vi "TestClone.vi"() -> ()   [LabVIEW 2014, in "WfrmModule.lvlib"]
uses:
  WfrmModule.lvlib
  WfrmPlugins/EventPluginBaseClass/TypeDefs/WfrmConfig.ctl
  PublicAPI/Arguments/Requests/dblEvtParams.ctl
  PublicAPI/Arguments/Requests/dblTimeArray.ctl
  WfrmPlugins/EventPluginBaseClass/TypeDefs/clEvtReportArray.ctl
  WfrmPlugins/EventPluginBaseClass/TypeDefs/clEvtReport.ctl
  WfrmPlugins/EventPluginBaseClass/TypeDefs/dblEvtSignalArray.ctl
  PublicAPI/Arguments/Requests/clTimeParams.ctl
  <userlib>/NIST/ModuleAdminLib/ModuleAdmin/ModuleAdmin.lvclass/ModuleAdmin.ctl
  <userlib>/NIST/ModuleAdminLib/ModuleAdmin/ModuleAdmin.lvclass
  WfrmPlugins/EventPluginBaseClass/TypeDefs/clWfrmParams.ctl
  PublicAPI/Arguments/Broadcasts/clDidInit.ctl
  PublicAPI/Arguments/Requests/clStopArgument.ctl
  <userlib>/NIST/ModuleAdminLib/ModuleAdmin/Accessors/Read CloneRegRef.vi
  <userlib>/NIST/ModuleAdminLib/ModuleAdmin/Accessors/Write CloneRegRef.vi
  <userlib>/NIST/ModuleAdminLib/CloneRegistration/CloneRegistration.lvclass
  WfrmPlugins/EventPluginBaseClass/BaseWfrmPlugin.lvclass
  <vilib>/Analysis/NI_AALBase.lvlib
  <vilib>/Analysis/1siggen.llb/Ramp Pattern by Delta.vi
panel:
  in  "btnConfigure":bool
  out "Settling Time":dbl
  in  "End Time":dbl=10.0
  in  "Start Time":dbl
  in  "WfrmParams":string[][](table)
  in  "Plugin Type":u16(ring) items=["C37.118.1", "HIL PMU", "60255Harm", "User1", "User2"]
  in  "clTimeParams":T1={"dblTimeArray"=[0.0, 0.05, 0.1, 0.15000000000000002, 0.2], "StartTime"=0.0, "EndTime"=1.0, "SettlingTime"=0.0}
  in  "btnSendArbWfrm":bool
  in  "btnGetEvtSignal":bool
  out "dblEventSignalArray":T2
  out "PathToPluginIniFileReport":path=path "P:/Framework/Events/EventPlugins/SSEvtPlugin/SteadyStateEventPlugin.ini"
  in  "btnReadPathToPlugin":bool
  in  "btnGetEvtReportArray":bool
  out "clEvtReportArray":T3 {"Synx" format="%#_4g"}
  in  "btnReadEvtParams":bool
  in  "btnWriteEvtParams":bool
  in  "btnReadTimeArray":bool
  in  "btnWriteTimeArray":bool
  out "dblTimeArrayReport":T5
  out "dblEvtParamsReport":T6
  in  "btnReadEvtConfig":bool
  in  "clEvtConfig":T7={"T0(UTC)"=0.0, "F0"=60.0, "Fs"=60, "FSamp"=960}
  in  "btnWriteEvtConfig":bool
  in  "btnLoadPlugin":bool
  in  "btnRemove":bool
  out "Status":string
  out "Active Modules (Array)":string[](array[string])
  in  "btnAdd":bool
  in  "btnStop":bool
  in  "Select Module":i32(ring)=-1 caption="Select Module to send Request" items=["All"=-1, "4140002"=4140002]
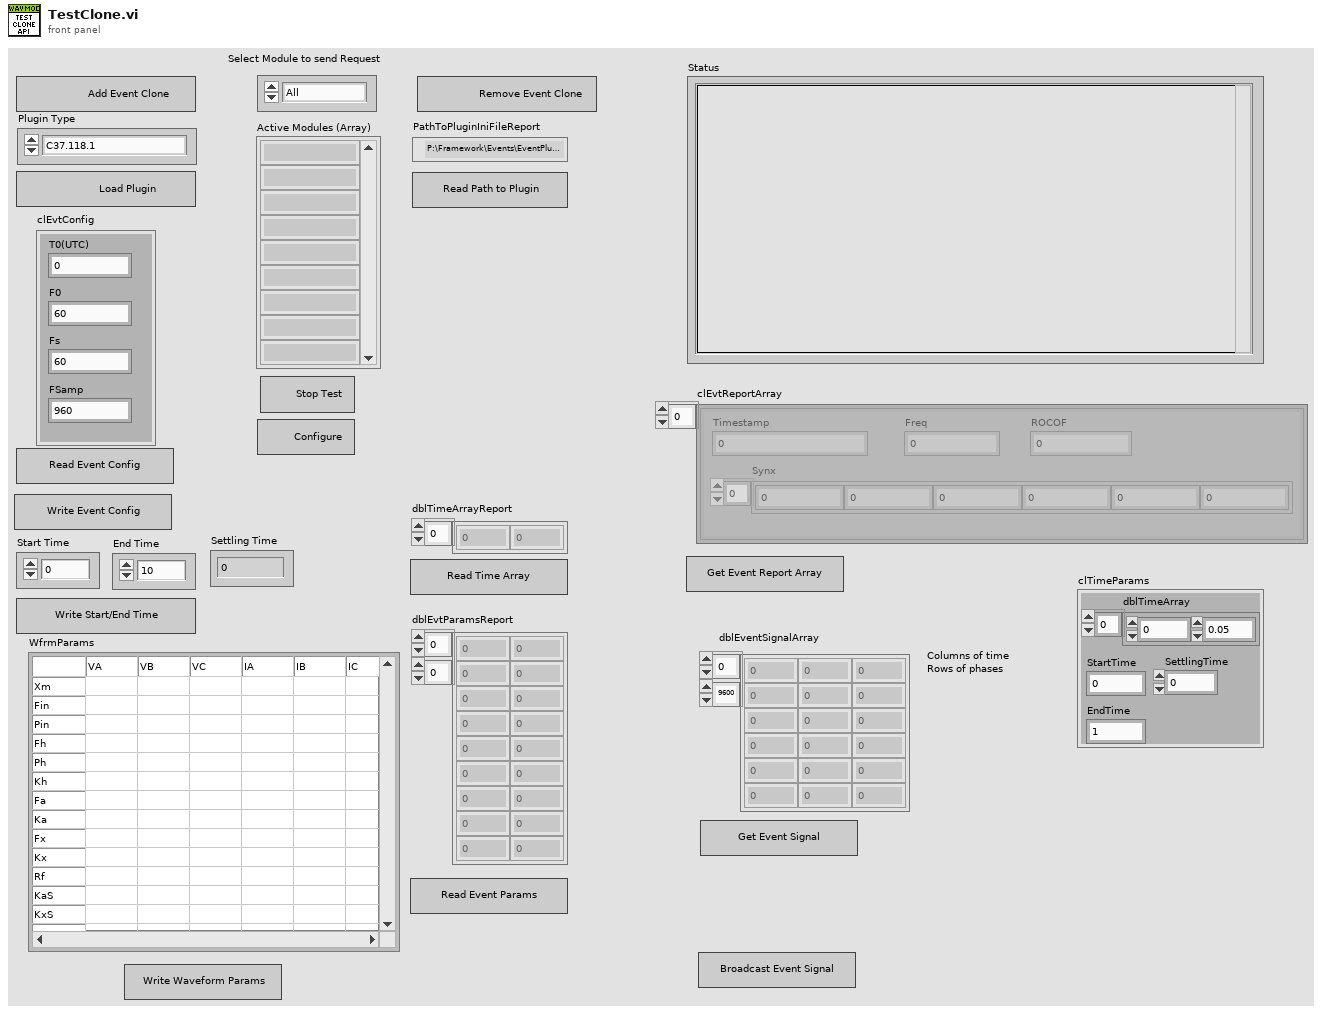
[diagram p1: front panel]
types:
  T1 = typedef "WfrmModule.lvlib/clTimeParams.ctl" = cluster{"dblTimeArray":dbl[], "StartTime":dbl, "EndTime":dbl, "SettlingTime":dbl}
  T2 = typedef "WfrmPlugins.lvlib/BaseWfrmPlugin.lvclass/dblEvtSignalArray.ctl" = dbl[][]
  T3 = typedef "WfrmPlugins.lvlib/BaseWfrmPlugin.lvclass/clEvtReportArray.ctl" = T4[]
  T4 = typedef "WfrmPlugins.lvlib/BaseWfrmPlugin.lvclass/clEvtReport.ctl" = cluster{"Timestamp":dbl, "Synx":cdb[], "Freq":dbl, "ROCOF":dbl}
  T5 = typedef "WfrmModule.lvlib/dblTimeArray.ctl" = dbl[]
  T6 = typedef "WfrmModule.lvlib/dblEvtParams.ctl" = dbl[][]
  T7 = typedef "WfrmPlugins.lvlib/BaseWfrmPlugin.lvclass/WfrmConfig.ctl" = cluster{"T0(UTC)":dbl, "F0":dbl, "Fs":i32, "FSamp":u32}
  T8 = typedef "WfrmModule.lvlib/clBroadcastEvents.ctl" = cluster{"DidInit":refnum<user-event>, "StatusUpdate":refnum<user-event>, "ErrorReport":refnum<user-event>, "DidStop":refnum<user-event>, "ReadEvtConfig":refnum<user-event>, "ReadTimeArray":refnum<user-event>, "ReadEvtParams":refnum<user-event>, "GetEvtReportArray":refnum<user-event>, "ReadPathToPlugin":refnum<user-event>, "GetEvtSignal":refnum<user-event>, "SendArbWfrm":refnum<user-event>, "WfrmParams":refnum<user-event>, "StartEndSettling":refnum<user-event>}
  T9 = typedef "WfrmPlugins.lvlib/BaseWfrmPlugin.lvclass/clWfrmParams.ctl" = cluster{"RowHdrs":string[], "ColHdrs":string[], "DefaultParams":string[][]}
  T10 = typedef "WfrmModule.lvlib/clDidInit.ctl" = cluster{"Init?":bool, "ModuleAdmin":refnum<class "ModuleAdmin.lvclass">}
  T11 = typedef "WfrmModule.lvlib/clStopArgument.ctl" = cluster{"Exit via Stop Module Req?":bool, "Wait for Module to stop?":bool, "ModuleAdmin":refnum<class "ModuleAdmin.lvclass">}
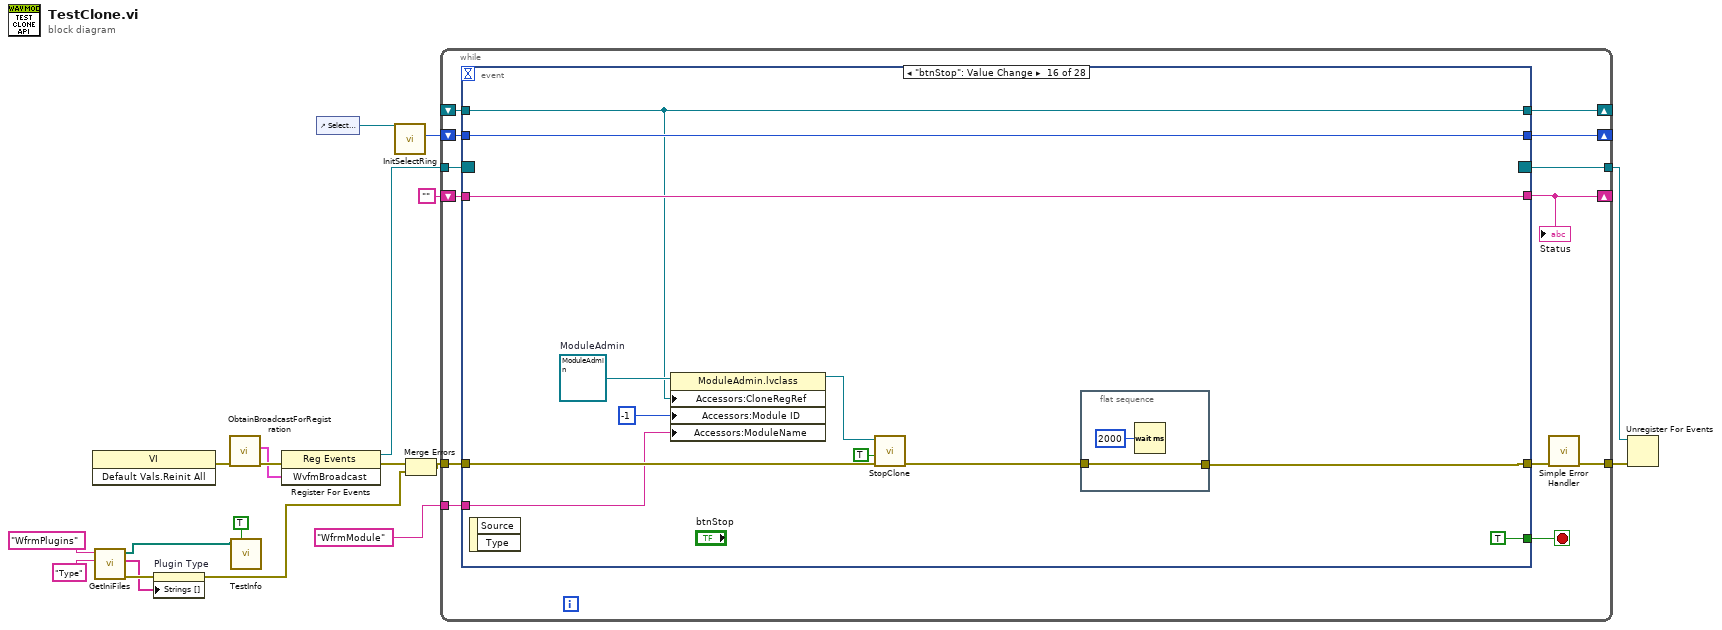
[diagram p0: block diagram]
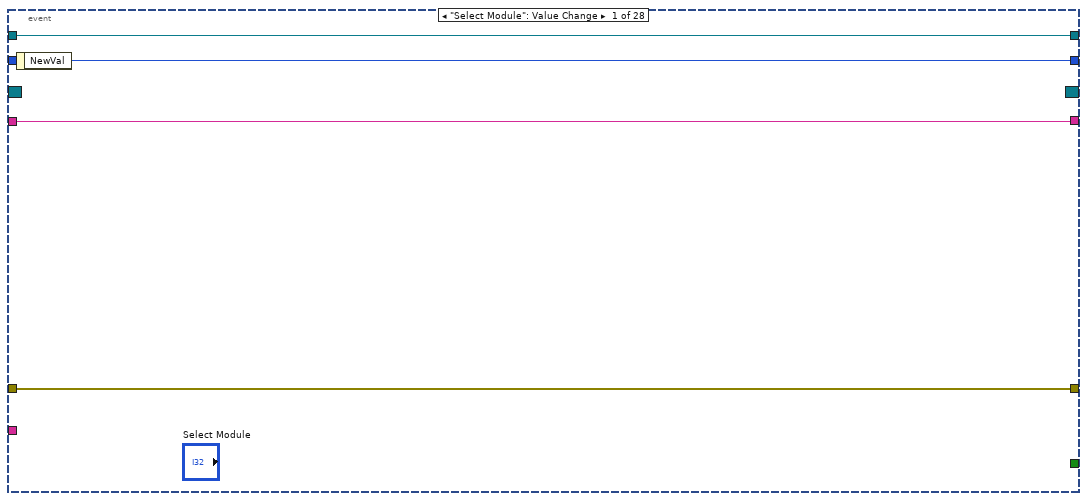
[diagram p2: hidden frame]
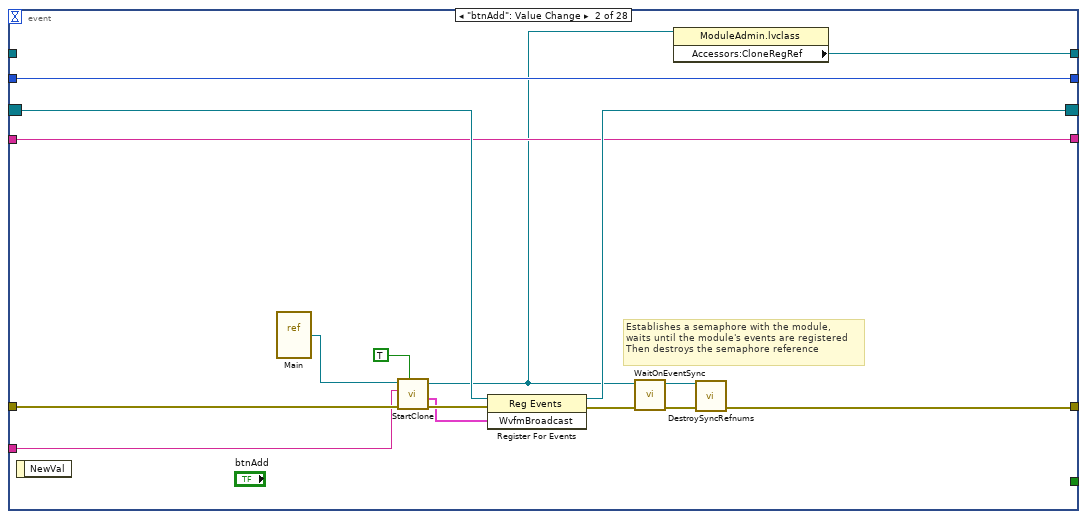
[diagram p3: hidden frame]
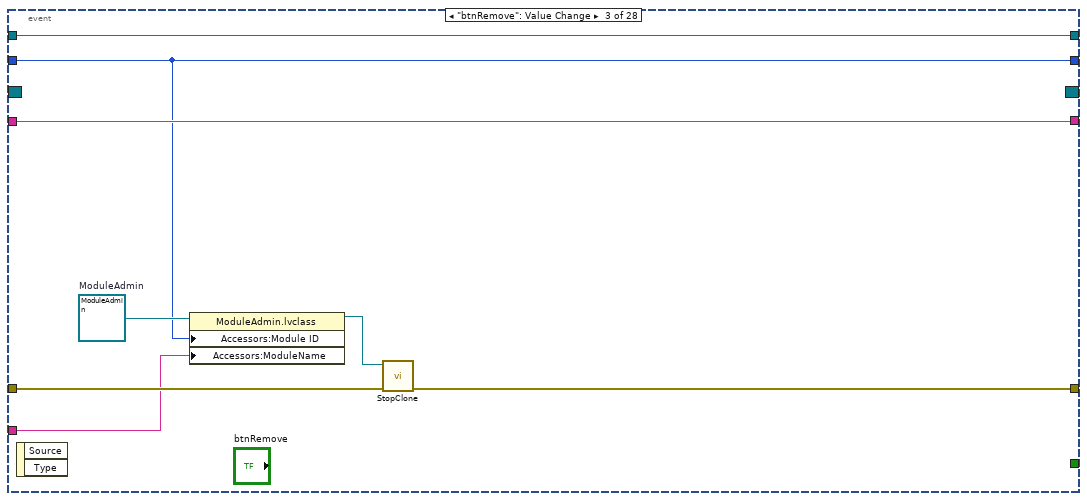
[diagram p4: hidden frame]
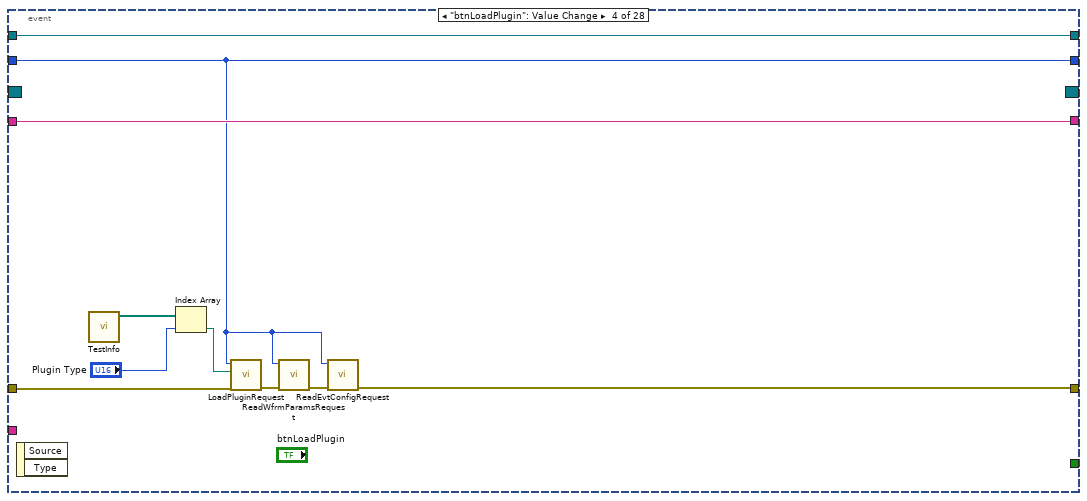
[diagram p5: hidden frame]
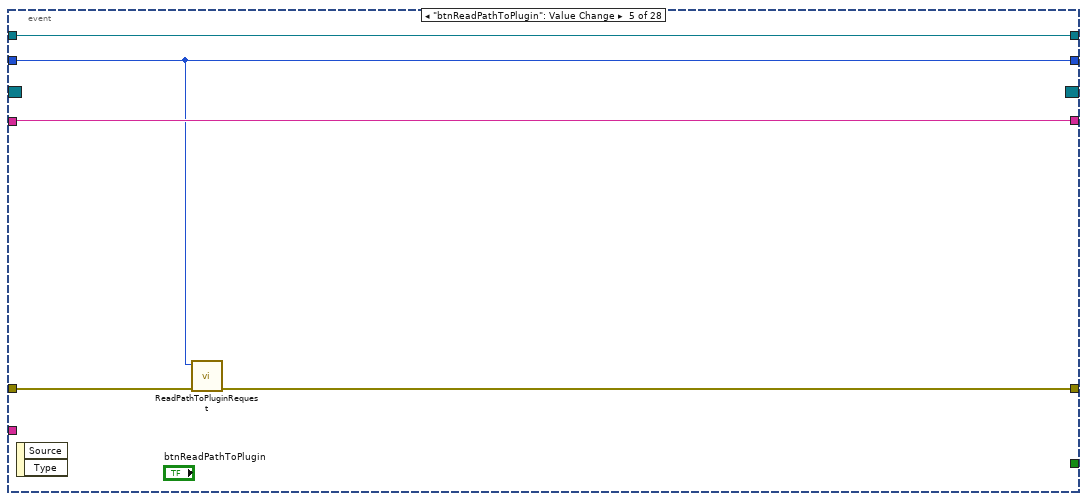
[diagram p6: hidden frame]
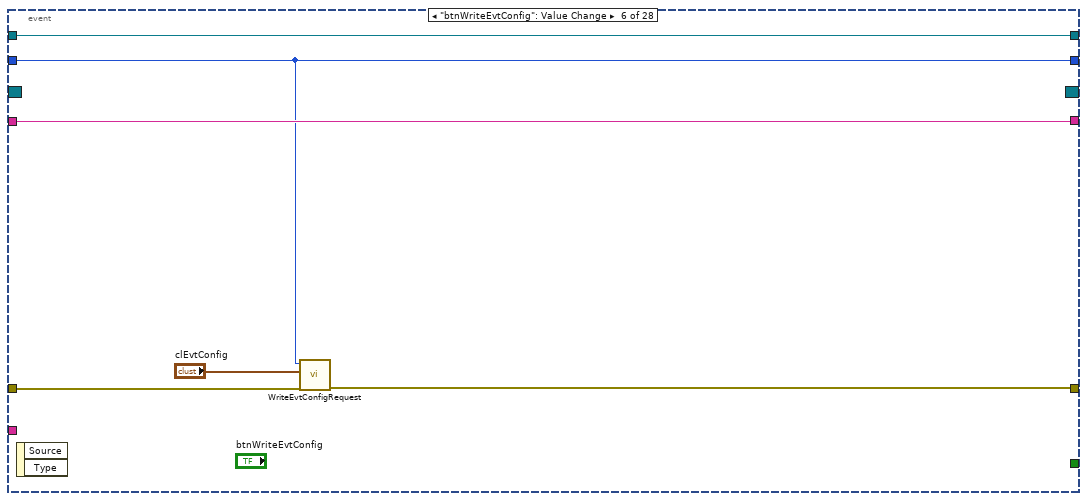
[diagram p7: hidden frame]
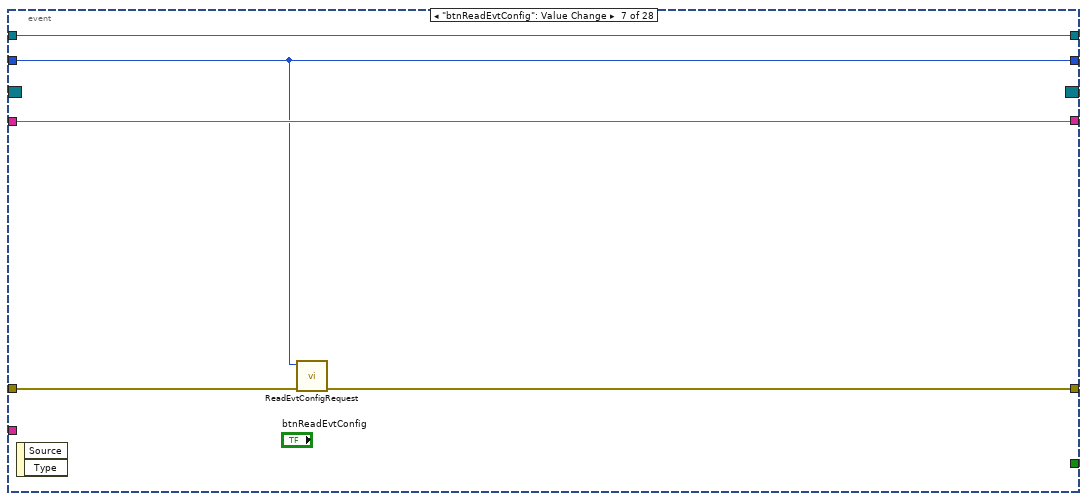
[diagram p8: hidden frame]
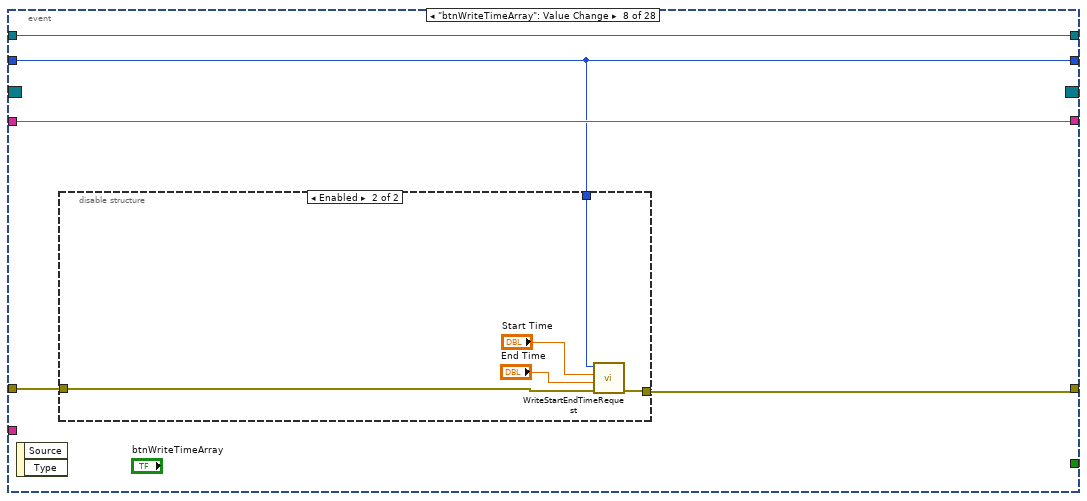
[diagram p9: hidden frame]
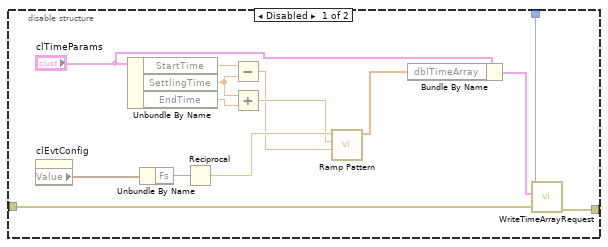
[diagram p10: hidden frame]
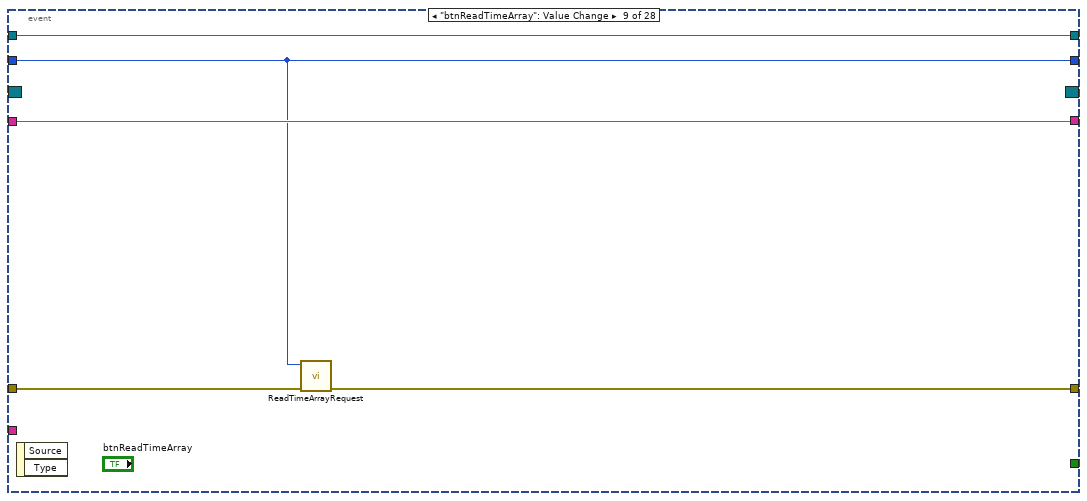
[diagram p11: hidden frame]
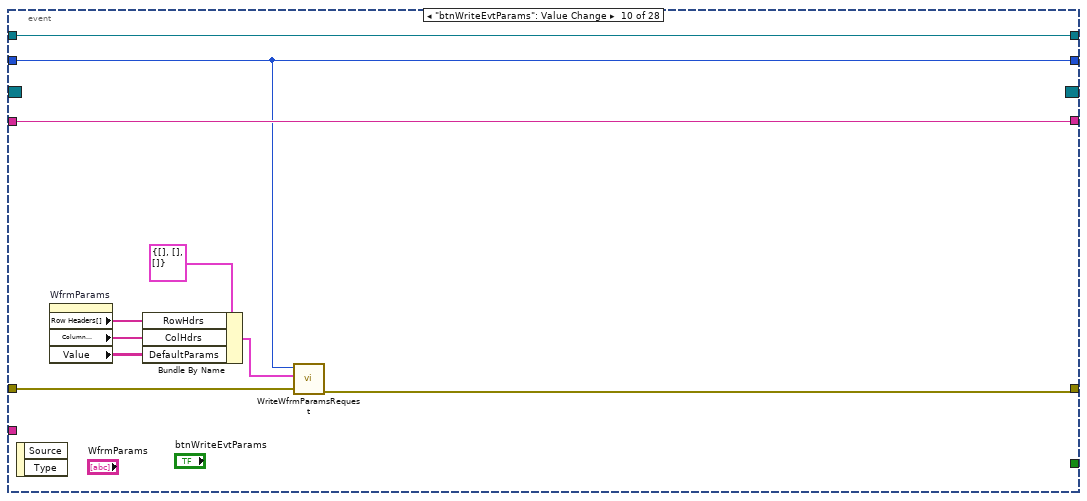
[diagram p12: hidden frame]
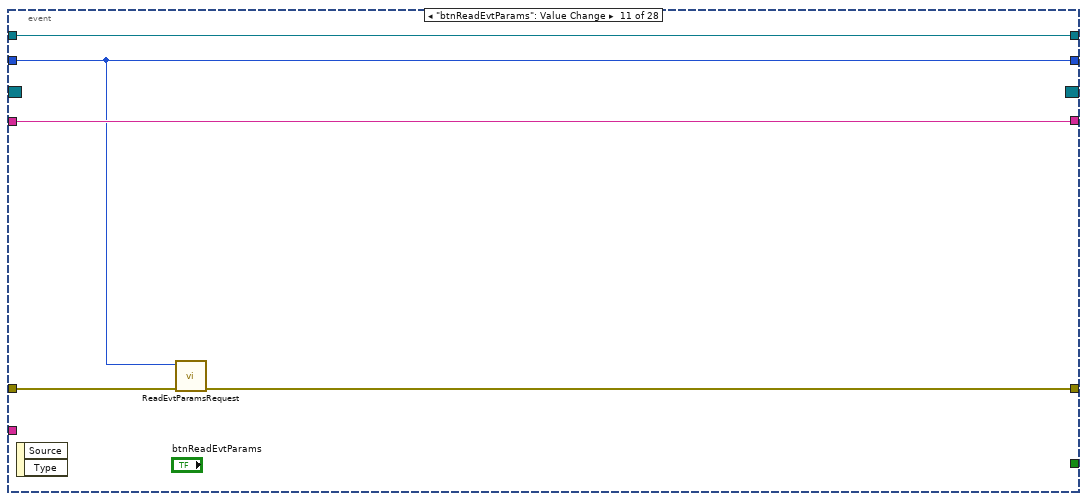
[diagram p13: hidden frame]
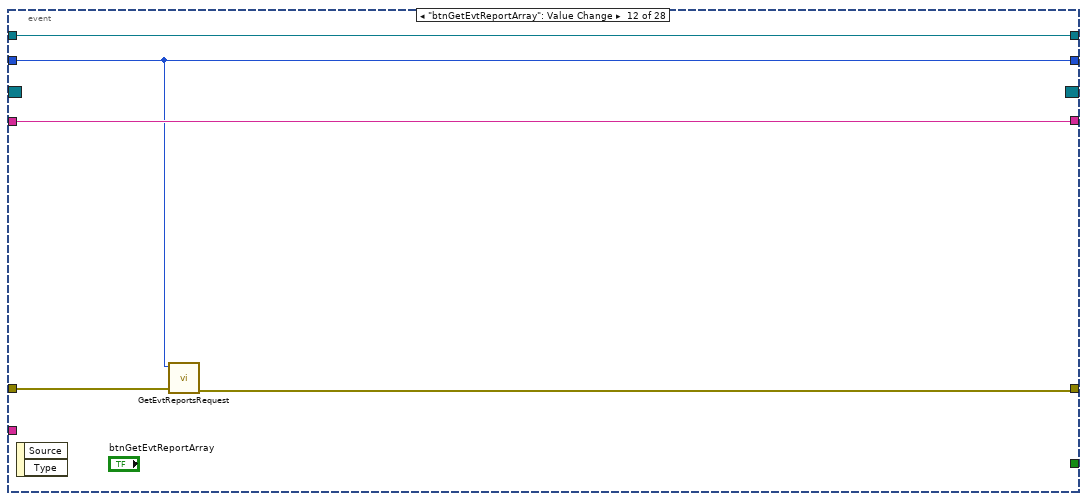
[diagram p14: hidden frame]
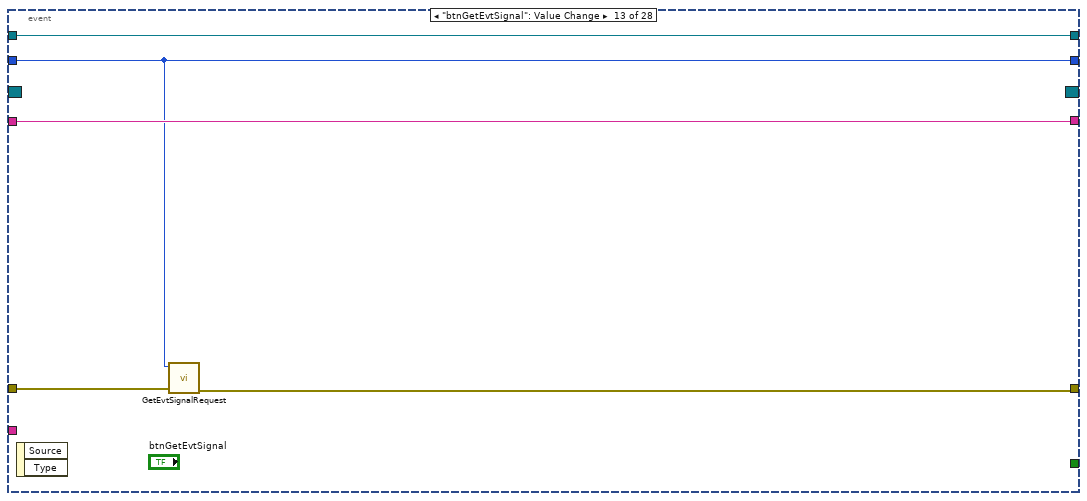
[diagram p15: hidden frame]
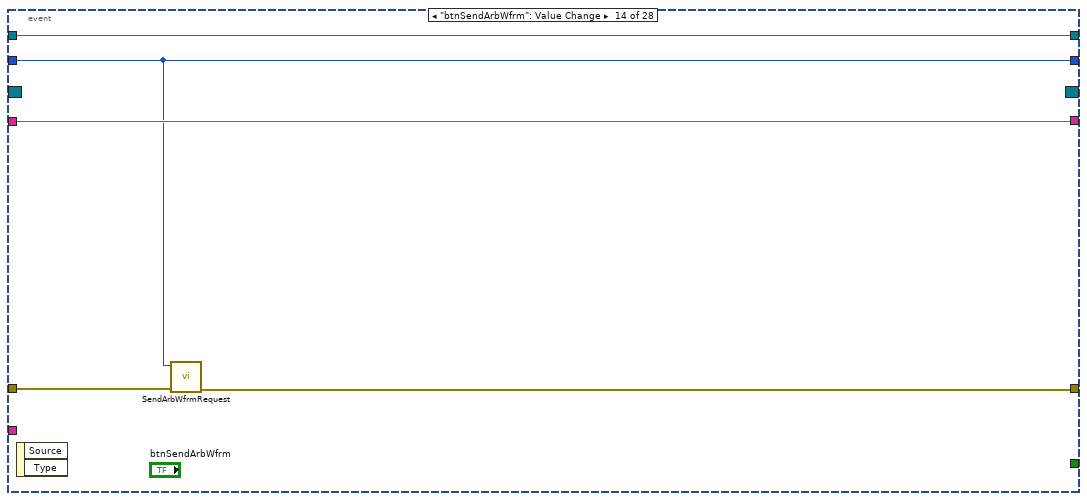
[diagram p16: hidden frame]
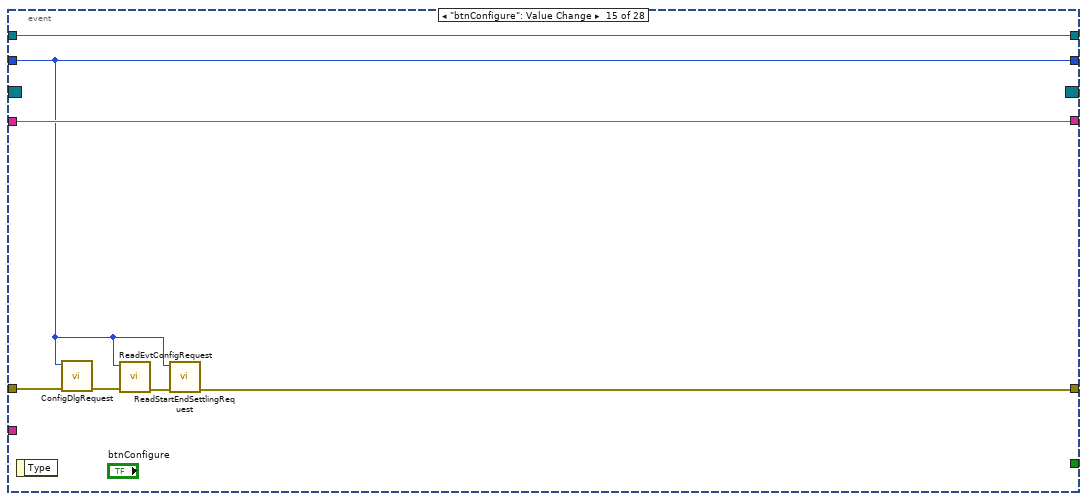
[diagram p17: hidden frame]
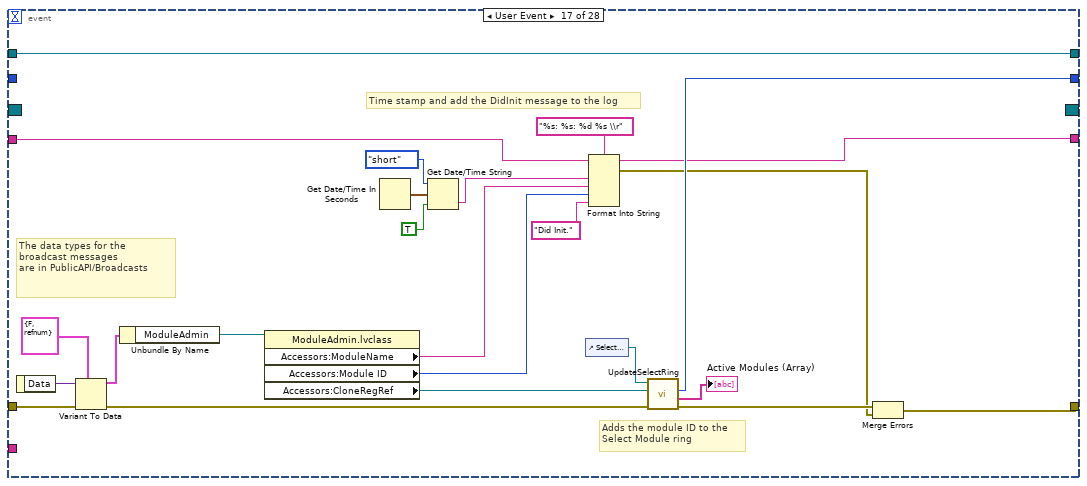
[diagram p18: hidden frame]
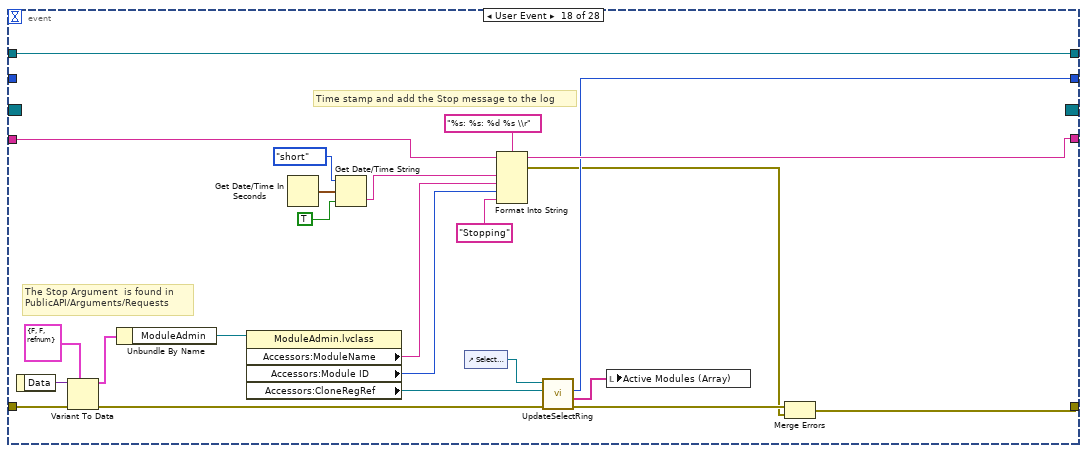
[diagram p19: hidden frame]
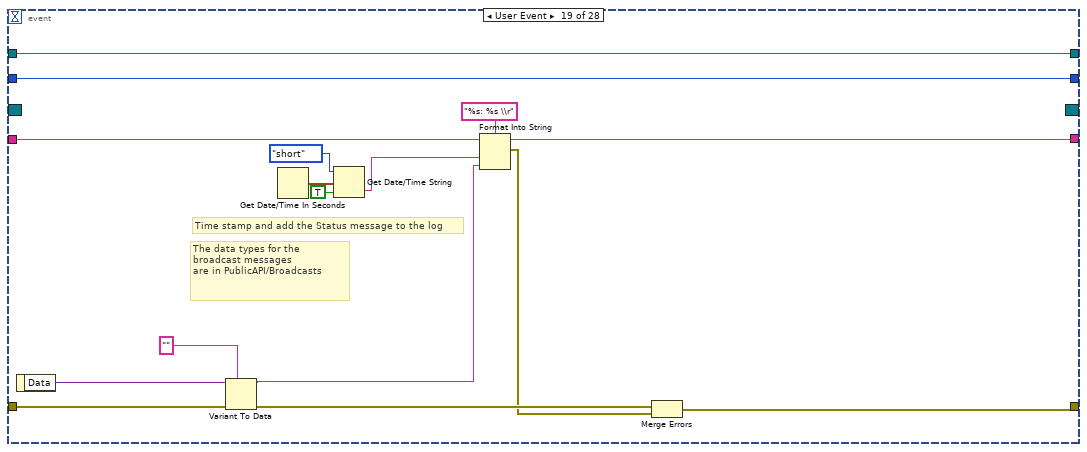
[diagram p20: hidden frame]
diagram:
  n1 = invoke class="VI" method="Default Vals.Reinit All"() -> (error out=w17:errorcluster)  [unwired: 3 in, 2 out]
  n2 = call "GetIniFiles.vi"("iniKey"="Type", "name or relative path"="WfrmPlugins") -> ("error out"=w10:errorcluster, "Types"=w9:string[], "IniFilePaths"=w5:path[])  [unwired: 7 in]
  n3 = property on="Plugin Type" class="Ring (strict)"(error in=w10, "Strings []"=w9) -> (error out=w7:errorcluster)  [unwired: 1 in, 1 out]
  n4 = call "ObtainBroadcastForRegistration.vi"("error in (no error)"=w17) -> ("error out"=w16:errorcluster, "WvfmBroadcast"=w15:T8)  [unwired: 9 in]
  n5 = call "TestInfo.vi"("Set (f)"=TRUE, "PluginIniFilePaths"=w5) -> ()  [unwired: 9 in, 1 out]
  n6 = register-events(error in=w16, w15) -> (reference out=w13:refnum<event-registration>, error out=w14:errorcluster)  [unwired: 1 in]
  n7 = control-ref of="Select Module"() -> (w19:refnum<vi>)
  n8 = call "InitSelectRing.vi"("Ring Refnum"=w19) -> ("Module Ring Value"=w18:i32)  [unwired: 9 in, 1 out]
  n9 = Merge Errors(w14, w7) -> (w8:errorcluster)
  n10 = while {
    shift-right: [w31] -> _
    shift-left: w18 -> [w32]
    tunnel: w8 -> [w29]
    tunnel: w13 -> [w26]
    tunnel: [w27] -> w2
    shift-right: [w25] -> _
    shift-left: "" -> [w24]
    tunnel: "WfrmModule" ("ModuleName") -> [w23]
    tunnel: [w22] -> w1
    shift-right: [w21] -> _
    shift-left: _ -> [w20]
    stop <- w30 stop-if-true
    n11 = event shown="[15] \"btnStop\": Value Change" {
      selector: w26 -> [_ w44 _ _ _ _ _ _ _ _ _ _ _ _ _ _ _ _ _ _ _ _ _ _ _ _ _ _]
      dyn-events: [_ w43 _ _ _ _ _ _ _ _ _ _ _ _ _ _ _ _ _ _ _ _ _ _ _ _ _ _] -> w22
      timeout: _ -> [_ _ _ _ _ _ _ _ _ _ _ _ _ _ _ _ _ _ _ _ _ _ _ _ _ _ _ _]
      tunnel: w32 -> [_ w52 w55 w61 w71 w77 w82 w87 w113 w121 w127 w131 w136 w141 w146 w163 _ _ w229 w234 w244 w251 w259 w266 w280 w287 w296 w312]
      tunnel: [w36 w52 w55 w61 w71 w77 w82 w87 w113 w121 w127 w131 w136 w141 w146 w163 w184 w200 w229 w234 w244 w251 w259 w266 w280 w287 w296 w312] -> w31
      tunnel: [_ _ _ _ _ _ _ _ _ _ _ _ _ _ _ TRUE _ _ _ _ _ _ _ _ _ _ _ _] -> w30
      tunnel: w29 -> [w34 w51 w59 w69 w73 w79 w84 w90 w112 w124 w128 w134 w139 w143 w151 w161 w189 w209 w226 w238 w246 w256 w261 w275 w283 w292 w300 w310]
      tunnel: [w34 w45 w58 w62 w72 w76 w83 w89 w111 w122 w126 w133 w138 w142 w145 w154 w172 w197 w220 w237 w240 w255 w262 w268 w282 w291 w299 w303] -> w28
      tunnel: [w35 w41 w60 w68 w74 w80 w85 w88 w114 w123 w129 w132 w137 w144 w149 w159 w176 w206 w223 w233 w245 w250 w260 w265 w281 w288 w297 w307] -> w25
      tunnel: w24 -> [w35 w41 w60 w68 w74 w80 w85 w88 w114 w123 w129 w132 w137 w144 w149 w159 w175 w207 w228 w233 w245 w250 w260 w265 w281 w288 w297 w307]
      tunnel: w23 -> [_ w40 w56 _ _ _ _ _ _ _ _ _ _ _ _ w157 _ _ _ _ _ _ _ _ _ _ _ _]
      tunnel: [w33 w37 w53 w64 w70 w75 w81 w86 w110 w120 w125 w130 w135 w140 w150 w152 w166 w190 w214 w230 w243 w249 w257 w267 w277 w285 w293 w313] -> w21
      tunnel: w20 -> [w33 _ w53 w64 w70 w75 w81 w86 w110 w120 w125 w130 w135 w140 w150 w152 w166 w190 w214 w230 w243 w249 w257 w267 w277 w285 w293 w313]
      event "Select Module": Value Change {
        n12 = event-data() -> ("NewVal"=w36:i32)  [unwired: 1 in]
      }
      event "btnAdd": Value Change {
        # "Establishes a semaphore with the module,\nwaits until the module's events are registered\nThen destroys the semaphore reference"
        n13 = event-data() -> ()  [unwired: 1 in, 1 out]
        n14 = vi-ref "Main.vi"() -> (w42:refnum<vi>)
        n15 = call "StartClone.vi"("ShowPanel? (F)"=TRUE, "error in (no error)"=w51, "ModuleName"=w40, "VI Refnum"=w42) -> ("error out"=w50:errorcluster, "WvfrmEvents"=w46:T8, "ModuleAdmin"=w38:refnum<class "ModuleAdmin.lvclass">)  [unwired: 5 in]
        n16 = register-events(reference=w44, error in=w50, w46) -> (reference out=w43:refnum<event-registration>, error out=w49:errorcluster)
        n17 = call <userlib>:"WaitOnEventSync.vi"("error in (no error)"=w49, "ModuleAdmin"=w38) -> ("error out"=w48:errorcluster, "ModuleAdmin"=w47:refnum<class "ModuleAdmin.lvclass">)  [unwired: 8 in]
        n18 = property class="ModuleAdmin.lvclass"(reference=w38) -> ("Accessors:CloneRegRef"=w37:refnum<data-value>)  [unwired: 1 in, 2 out]
        n19 = call <userlib>:"DestroySyncRefnums.vi"("error in (no error)"=w48, "ModuleAdmin"=w47) -> ("error out"=w45:errorcluster)  [unwired: 9 in]
      }
      event "btnRemove": Value Change {
        w57 = refnum<class "ModuleAdmin.lvclass"> refnum  # ModuleAdmin
        n20 = event-data() -> ()  [unwired: 1 in, 2 out]
        n21 = property class="ModuleAdmin.lvclass"(reference=w57, "Accessors:Module ID"=w55, "Accessors:ModuleName"=w56) -> (reference out=w54:refnum<class "ModuleAdmin.lvclass">)  [unwired: 1 in, 1 out]
        n22 = call "StopClone.vi"("error in (no error)"=w59, "ModuleAdmin"=w54) -> ("error out"=w58:errorcluster)  [unwired: 9 in]
      }
      event "btnLoadPlugin": Value Change {
        n23 = event-data() -> ()  [unwired: 1 in, 2 out]
        n24 = call "TestInfo.vi"() -> ("PluginIniFilePaths"=w67:path[])  [unwired: 11 in]
        n25 = Index Array(array=w67, index="Plugin Type") -> (element=w65:path)
        n26 = call "LoadPluginRequest.vi"("error in (no error)"=w69, "PathToPlugin"=w65, "ModuleID"=w61) -> ("error out"=w63:errorcluster)  [unwired: 8 in]
        n27 = call "ReadWfrmParamsRequest.vi"("error in (no error)"=w63, "ModuleID"=w61) -> ("error out"=w62:errorcluster)  [unwired: 9 in]
        n28 = call "ReadEvtConfigRequest.vi"("error in (no error)"=w62, "ModuleID"=w61) -> ()  [unwired: 9 in, 1 out]
      }
      event "btnReadPathToPlugin": Value Change {
        n29 = event-data() -> ()  [unwired: 1 in, 2 out]
        n30 = call "ReadPathToPluginRequest.vi"("error in (no error)"=w73, "ModuleID"=w71) -> ("error out"=w72:errorcluster)  [unwired: 9 in]
      }
      event "btnWriteEvtConfig": Value Change {
        n31 = event-data() -> ()  [unwired: 1 in, 2 out]
        n32 = call "WriteEvtConfigRequest.vi"("error in (no error)"=w79, "clEvtConfig"="clEvtConfig", "ModuleID"=w77) -> ("error out"=w76:errorcluster)  [unwired: 8 in]
      }
      event "btnReadEvtConfig": Value Change {
        n33 = event-data() -> ()  [unwired: 1 in, 2 out]
        n34 = call "ReadEvtConfigRequest.vi"("error in (no error)"=w84, "ModuleID"=w82) -> ("error out"=w83:errorcluster)  [unwired: 9 in]
      }
      event "btnWriteTimeArray": Value Change {
        n35 = event-data() -> ()  [unwired: 1 in, 2 out]
        n36 = disable-structure shown="Enabled" {
          disable-tunnel: w90 -> [w104 w109]
          disable-tunnel: [w103 w108] -> w89
          disable-tunnel: w87 -> [w102 w106]
          frame Disabled {
            n37 = property on="clEvtConfig" class="Clust (strict)"() -> ("Value"=w101:T7)  [unwired: 2 in, 2 out]
            n38 = Unbundle By Name("clTimeParams") -> ("StartTime"=w98:dbl, "SettlingTime"=w97:dbl, "EndTime"=w96:dbl)
            n39 = Unbundle By Name(w101) -> ("Fs"=w100:i32)
            n40 = Reciprocal(x=w100) -> (1/x=w99:dbl)
            n41 = Subtract(x=w98, y=w97) -> (x-y=w94:dbl)
            n42 = Add(x=w97, y=w96) -> (x+y=w95:dbl)
            n43 = call-poly <vilib>:"Ramp Pattern.vi"("start"=w94, "end"=w95, "delta"=w99) -> ("Ramp Pattern"=w92:dbl[])  [unwired: 6 in, 2 out]
            n44 = Bundle By Name(cluster="clTimeParams", "dblTimeArray"=w92) -> (w91:T1)
            n45 = call "WriteTimeArrayRequest.vi"("error in (no error)"=w104, "clTimeParams"=w91, "ModuleID"=w102) -> ("error out"=w103:errorcluster)  [unwired: 8 in]
          }
          frame Enabled {
            n46 = call "WriteStartEndTimeRequest.vi"("error in (no error)"=w109, "EndTime"="End Time", "StartTime"="Start Time", "ModuleID"=w106) -> ("error out"=w108:errorcluster)  [unwired: 7 in]
          }
        }
      }
      event "btnReadTimeArray": Value Change {
        n47 = event-data() -> ()  [unwired: 1 in, 2 out]
        n48 = call "ReadTimeArrayRequest.vi"("error in (no error)"=w112, "ModuleID"=w113) -> ("error out"=w111:errorcluster)  [unwired: 9 in]
      }
      event "btnWriteEvtParams": Value Change {
        n49 = event-data() -> ()  [unwired: 1 in, 2 out]
        n50 = property on="WfrmParams" class="Tbl (strict)"() -> ("Row Headers[]"=w118:string[], "Column Headers[]"=w117:string[], "Value"=w116:string[][])  [unwired: 2 in, 2 out]
        n51 = Bundle By Name(cluster=T9 {"RowHdrs"=[], "ColHdrs"=[], "DefaultParams"=[]} ("clWfrmParams"), "RowHdrs"=w118, "ColHdrs"=w117, "DefaultParams"=w116) -> (w115:T9)
        n52 = call "WriteWfrmParamsRequest.vi"("error in (no error)"=w124, "WfrmParams"=w115, "ModuleID"=w121) -> ("error out"=w122:errorcluster)  [unwired: 8 in]
      }
      event "btnReadEvtParams": Value Change {
        n53 = event-data() -> ()  [unwired: 1 in, 2 out]
        n54 = call "ReadEvtParamsRequest.vi"("error in (no error)"=w128, "ModuleID"=w127) -> ("error out"=w126:errorcluster)  [unwired: 9 in]
      }
      event "btnGetEvtReportArray": Value Change {
        n55 = event-data() -> ()  [unwired: 1 in, 2 out]
        n56 = call "GetEvtReportsRequest.vi"("error in (no error)"=w134, "ModuleID"=w131) -> ("error out"=w133:errorcluster)  [unwired: 9 in]
      }
      event "btnGetEvtSignal": Value Change {
        n57 = event-data() -> ()  [unwired: 1 in, 2 out]
        n58 = call "GetEvtSignalRequest.vi"("error in (no error)"=w139, "ModuleID"=w136) -> ("error out"=w138:errorcluster)  [unwired: 9 in]
      }
      event "btnSendArbWfrm": Value Change {
        n59 = event-data() -> ()  [unwired: 1 in, 2 out]
        n60 = call "SendArbWfrmRequest.vi"("error in (no error)"=w143, "ModuleID"=w141) -> ("error out"=w142:errorcluster)  [unwired: 9 in]
      }
      event "btnConfigure": Value Change {
        n61 = event-data() -> ()  [unwired: 1 in, 1 out]
        n62 = call "ConfigDlgRequest.vi"("error in (no error)"=w151, "ModuleID"=w146) -> ("error out"=w148:errorcluster)  [unwired: 9 in]
        n63 = call "ReadEvtConfigRequest.vi"("error in (no error)"=w148, "ModuleID"=w146) -> ("error out"=w147:errorcluster)  [unwired: 9 in]
        n64 = call "ReadStartEndSettlingRequest.vi"("error in (no error)"=w147, "ModuleID"=w146) -> ("error out"=w145:errorcluster)  [unwired: 9 in]
      }
      event "btnStop": Value Change {
        w158 = refnum<class "ModuleAdmin.lvclass"> refnum  # ModuleAdmin
        n65 = event-data() -> ()  [unwired: 1 in, 2 out]
        n66 = property class="ModuleAdmin.lvclass"(reference=w158, "Accessors:CloneRegRef"=w152, "Accessors:Module ID"=-1 ("Module ID"), "Accessors:ModuleName"=w157) -> (reference out=w156:refnum<class "ModuleAdmin.lvclass">)  [unwired: 1 in, 1 out]
        n67 = call "StopClone.vi"("error in (no error)"=w161, "Wait for Module to stop?"=TRUE, "ModuleAdmin"=w156) -> ("error out"=w155:errorcluster)  [unwired: 8 in]
        n68 = flat-sequence {
          tunnel: [w164] -> w154
          tunnel: w155 -> [w164]
          frame #0 {
            n69 = Wait (ms)(milliseconds to wait=u32 2000) -> ()  [unwired: 1 out]
          }
        }
      }
      event User Event {
        # "Adds the module ID to the \nSelect Module ring"
        # "Time stamp and add the DidInit message to the log"
        # "The data types for the broadcast messages\nare in PublicAPI/Broadcasts"
        n70 = event-data() -> ("Data"=w188:variant)  [unwired: 1 in]
        n71 = Variant To Data(error in=w189, type=T10 {"Init?"=FALSE, "ModuleAdmin"=refnum} ("clDidInit"), Variant=w188) -> (data=w181:T10, error out=w186:errorcluster)
        n72 = Unbundle By Name(w181) -> ("ModuleAdmin"=w180:refnum<class "ModuleAdmin.lvclass">)
        n73 = property class="ModuleAdmin.lvclass"(reference=w180) -> ("Accessors:ModuleName"=w169:string, "Accessors:Module ID"=w168:i32, "Accessors:CloneRegRef"=w167:refnum<data-value>)  [unwired: 1 in, 2 out]
        n74 = Get Date/Time In Seconds() -> (seconds since 1Jan1904=w178:timestamp)
        n75 = Get Date/Time String(date format (0)=enum16{"short", "long", "abbreviated"}."short", seconds (now)=w178, want seconds? (F)=TRUE) -> (time string=w182:string)  [unwired: 1 out]
        n76 = control-ref of="Select Module"() -> (w185:refnum<vi>)
        n77 = Format Into String(format string="%s: %s: %d %s \\r", initial string=w175, w182, w169, w168, "Did Init.") -> (resulting string=w176:string, error out=w173:errorcluster)  [unwired: 1 in]
        n78 = call "UpdateSelectRing.vi"("error in (no error)"=w186, "CloneRegRef"=w167, "Ring Refnum"=w185) -> ("error out"=w174:errorcluster, "ActiveModules"=→"Active Modules (Array)":string[], "Module Ring Value"=w184:i32)  [unwired: 6 in]
        n79 = Merge Errors(w174, w173) -> (w172:errorcluster)
      }
      event User Event {
        # "Time stamp and add the Stop message to the log"
        # "The Stop Argument  is found in\nPublicAPI/Arguments/Requests"
        n80 = event-data() -> ("Data"=w208:variant)  [unwired: 1 in]
        n81 = Variant To Data(error in=w209, type=T11 {"Exit via Stop Module Req?"=FALSE, "Wait for Module to stop?"=FALSE, "ModuleAdmin"=refnum} ("Stop Argument"), Variant=w208) -> (data=w204:T11, error out=w203:errorcluster)
        n82 = Unbundle By Name(w204) -> ("ModuleAdmin"=w195:refnum<class "ModuleAdmin.lvclass">)
        n83 = property class="ModuleAdmin.lvclass"(reference=w195) -> ("Accessors:ModuleName"=w192:string, "Accessors:Module ID"=w191:i32, "Accessors:CloneRegRef"=w194:refnum<data-value>)  [unwired: 1 in, 2 out]
        n84 = Get Date/Time In Seconds() -> (seconds since 1Jan1904=w211:timestamp)
        n85 = Get Date/Time String(date format (0)=enum16{"short", "long", "abbreviated"}."short", seconds (now)=w211, want seconds? (F)=TRUE) -> (time string=w213:string)  [unwired: 1 out]
        n86 = control-ref of="Select Module"() -> (w202:refnum<vi>)
        n87 = Format Into String(format string="%s: %s: %d %s \\r", initial string=w207, w213, w192, w191, "Stopping") -> (resulting string=w206:string, error out=w198:errorcluster)  [unwired: 1 in]
        n88 = call "UpdateSelectRing.vi"("error in (no error)"=w203, "CloneRegRef"=w194, "Ring Refnum"=w202) -> ("error out"=w199:errorcluster, "ActiveModules"=w201:string[], "Module Ring Value"=w200:i32)  [unwired: 6 in]
        n89 = local write "Active Modules (Array)"(w201) -> ()
        n90 = Merge Errors(w199, w198) -> (w197:errorcluster)
      }
      event User Event {
        # "Time stamp and add the Status message to the log"
        # "The data types for the broadcast messages\nare in PublicAPI/Broadcasts"
        n91 = event-data() -> ("Data"=w225:variant)  [unwired: 1 in]
        n92 = Variant To Data(error in=w226, type="", Variant=w225) -> (data=w215:string, error out=w222:errorcluster)
        n93 = Get Date/Time In Seconds() -> (seconds since 1Jan1904=w224:timestamp)
        n94 = Get Date/Time String(date format (0)=enum16{"short", "long", "abbreviated"}."short", seconds (now)=w224, want seconds? (F)=TRUE) -> (time string=w217:string)  [unwired: 1 out]
        n95 = Format Into String(format string="%s: %s \\r", initial string=w228, w217, w215) -> (resulting string=w223:string, error out=w221:errorcluster)  [unwired: 1 in]
        n96 = Merge Errors(w222, w221) -> (w220:errorcluster)
      }
      event User Event {
        # "#CodeNeeded\nThis is a very crude error handler\nA better error handler will be needed"
        # "The data types for the broadcast messages\nare in PublicAPI/Broadcasts"
        n97 = event-data() -> ("ModuleID"=w236:i32, "Data"=w239:variant)  [unwired: 1 in]
        n98 = Variant To Data(error in=w238, type=errorcluster {"status"=FALSE, "code"=0, "source"=""} ("error constant"), Variant=w239) -> (data=w231:errorcluster, error out=w237:errorcluster)
        n99 = Number To Decimal String(number=w236) -> (decimal integer string=w235:string)  [unwired: 1 in]
        n100 = call <vilib>:"General Error Handler.vi"("[error source] (\" \")"=w235, "error in (no error)"=w231) -> ()  [unwired: 9 in, 5 out]
      }
      event User Event {
        n101 = event-data() -> ("Data"=w248:variant)  [unwired: 1 in]
        n102 = Variant To Data(error in=w246, type=T7 {"T0(UTC)"=0.0, "F0"=0.0, "Fs"=0, "FSamp"=0} ("clEvtConfig"), Variant=w248) -> (data=w242:T7, error out=w241:errorcluster)
        n103 = property on="clEvtConfig" class="Clust (strict)"(error in=w241, "Value"=w242) -> (error out=w240:errorcluster)  [unwired: 1 in, 1 out]
      }
      event User Event {
        w252 = T5 []  # TimeArray
        n104 = event-data() -> ("Data"=w253:variant)  [unwired: 1 in]
        n105 = Variant To Data(error in=w256, type=w252, Variant=w253) -> (data=→"dblTimeArrayReport":T5, error out=w255:errorcluster)
      }
      event User Event {
        w264 = T6 []  # SignalParams
        n106 = event-data() -> ("Data"=w258:variant)  [unwired: 1 in]
        n107 = Variant To Data(error in=w261, type=w264, Variant=w258) -> (data=→"dblEvtParamsReport":T6, error out=w262:errorcluster)
      }
      event User Event {
        n108 = event-data() -> ("Data"=w276:variant)  [unwired: 1 in, 1 out]
        n109 = Variant To Data(error in=w275, type=T9 {"RowHdrs"=[], "ColHdrs"=[], "DefaultParams"=[]} ("clWfrmParams"), Variant=w276) -> (data=w273:T9, error out=w272:errorcluster)
        n110 = Unbundle By Name(w273) -> ("RowHdrs"=w269:string[], "ColHdrs"=w270:string[], "DefaultParams"=w271:string[][])
        n111 = property on="WfrmParams" class="Tbl (strict)"(error in=w272, "Row Headers[]"=w269, "Column Headers[]"=w270, "Value"=w271) -> (error out=w268:errorcluster)  [unwired: 1 in, 1 out]
      }
      event User Event {
        n112 = event-data() -> ("Data"=w284:variant)  [unwired: 1 in]
        n113 = Variant To Data(error in=w283, type=path "", Variant=w284) -> (data=→"PathToPluginIniFileReport":path, error out=w282:errorcluster)
      }
      event User Event {
        w286 = T3 []  # ReportArray
        n114 = event-data() -> ("Data"=w290:variant)  [unwired: 1 in]
        n115 = Variant To Data(error in=w292, type=w286, Variant=w290) -> (data=→"clEvtReportArray":T3, error out=w291:errorcluster)
      }
      event User Event {
        n116 = event-data() -> ("Data"=w298:variant)  [unwired: 1 in]
        n117 = Variant To Data(error in=w300, type=T2 [] ("dblEventSignalArray"), Variant=w298) -> (data=→"dblEventSignalArray":T2, error out=w299:errorcluster)
      }
      event User Event {
        n118 = event-data() -> ("Data"=w311:variant)  [unwired: 1 in]
        n119 = Variant To Data(error in=w310, type=dbl[] [], Variant=w311) -> (data=w308:dbl[], error out=w305:errorcluster)
        n120 = Index Array(array=w308) -> (element #1=w301:dbl, element #2=w302:dbl, element #3=→"Settling Time":dbl)  [unwired: 3 in]
        n121 = property on="End Time" class="DigNum (strict)"(error in=w305, "Value"=w302) -> (error out=w304:errorcluster)  [unwired: 1 in, 1 out]
        n122 = property on="Start Time" class="DigNum (strict)"(error in=w304, "Value"=w301) -> (error out=w303:errorcluster)  [unwired: 1 in, 1 out]
      }
    }
    "Status" <- w25
    n123 = call <vilib>:"Simple Error Handler.vi"("error in (no error)"=w28) -> ("error out"=w27:errorcluster)  [unwired: 4 in, 4 out]
  }
  n124 = Unregister For Events(event registration refnum=w1, error in=w2) -> ()  [unwired: 1 out]
